vi "Push.vi"(8 "error in":errorcluster, 10 "IMessage":refnum<class "CAN Message.lvclass">, 11 "Message Buffer in":refnum<class "Message Buffer.lvclass">) -> (0 "error out":errorcluster, 3 "Message Buffer out":refnum<class "Message Buffer.lvclass">)   [LabVIEW 2024, in "PCAN.lvlib" / "Message Buffer.lvclass"]
uses:
  Message Buffer.lvclass
  Message Buffer.lvclass/Message Buffer.ctl
  CAN Message/CAN Message.lvclass
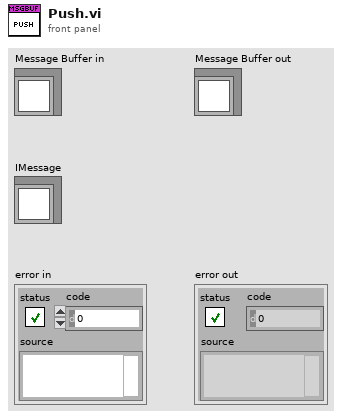
[diagram p1: front panel]
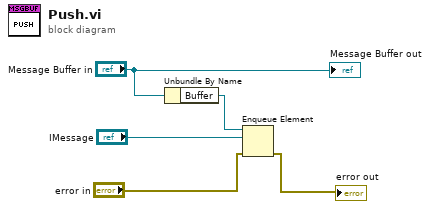
[diagram p0: block diagram]
diagram:
  n1 = Unbundle By Name("Message Buffer in") -> ("Buffer"=w1:refnum<queue>)
  n2 = Enqueue Element(queue=w1, element="IMessage", error in (no error)="error in") -> (error out=→"error out":errorcluster)  [unwired: 1 in, 2 out]
  "Message Buffer out" <- "Message Buffer in"
